vi "Calculate differential torque disproportion.vi"(8 "Error In":errorcluster, 10 "Steering (-123,123)":dbl[unit] format="%#_13g") -> (0 "Error Out":errorcluster, 1 "Right wheel diff scaller":dbl, 2 "Left wheel diff scaller":dbl)   [LabVIEW 2016]
panel:
  out "Right wheel R":dbl[unit]
  out "Left wheel R":dbl[unit]
  out "R xaxis":dbl[unit]
  out "Steer Angle":dbl[unit]
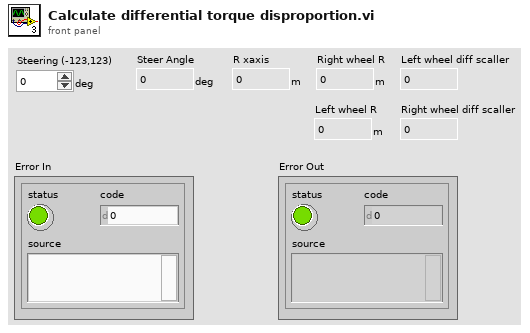
[diagram p1: front panel]
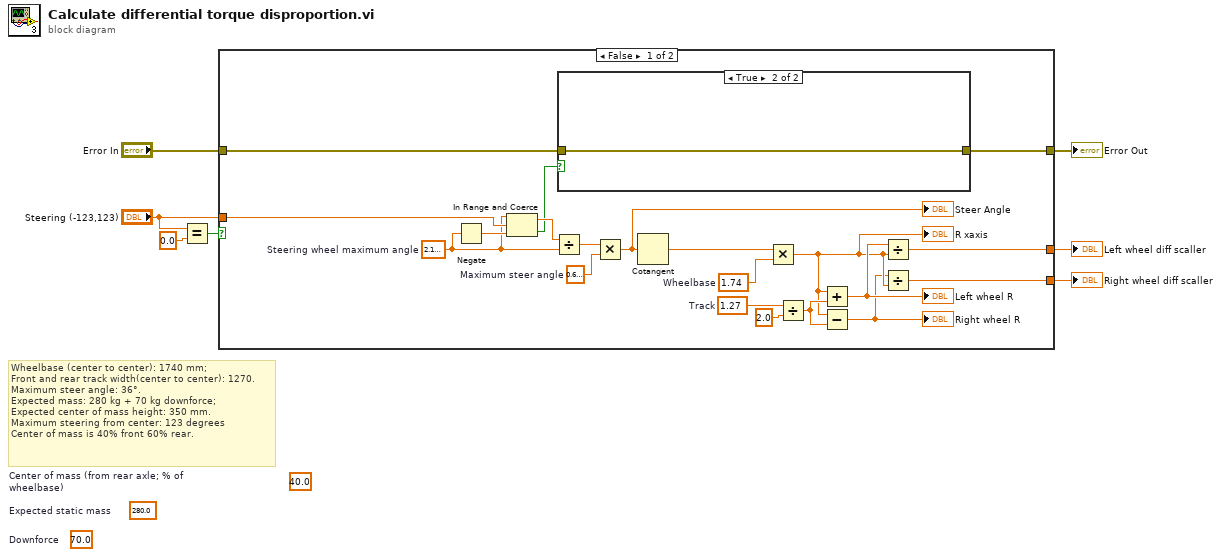
[diagram p0: block diagram]
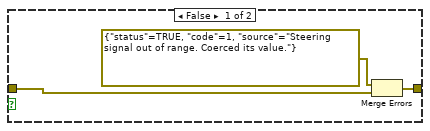
[diagram p2: hidden frame]
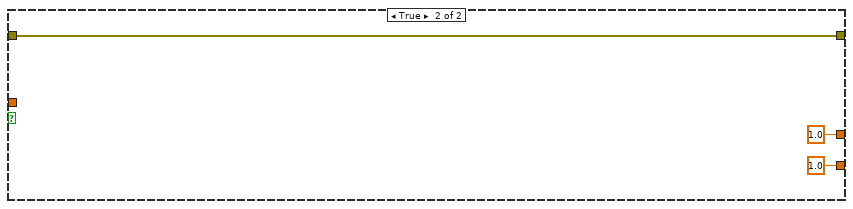
[diagram p3: hidden frame]
diagram:
  (unwired) dbl[unit] 40.0  # Center of mass (from rear axle; % of wheelbase)
  (unwired) dbl[unit] 70.0  # Downforce
  (unwired) dbl[unit] 280.0  # Expected static mass
  # "Wheelbase (center to center): 1740 mm; \nFront and rear track width(center to center): 1270. \nMaximum steer angle: 36°. \nExpected mass: 280 kg + 70 kg downforce; \nExpected center of mass height: 350 mm.\nMaximum steering from center: 123 degrees\nCenter of mass is 40% front 60% rear."
  n1 = Equal?(x="Steering (-123,123)", y=dbl[unit] 0.0) -> (x = y?=w7:bool)
  n2 = case shown="False" w7 {
    tunnel: "Steering (-123,123)" -> [w22 _]
    tunnel: [w24 1.0] -> w4
    tunnel: [w23 1.0] -> w3
    tunnel: "Error In" -> [w9 w32]
    tunnel: [w8 w32] -> w1
    frame False {
      w25 = dbl[unit] 1.27  # Track
      w26 = dbl[unit] 1.74  # Wheelbase
      w27 = dbl[unit] 0.6283185307179586  # Maximum steer angle
      w20 = dbl[unit] 2.1642082724729685  # Steering wheel maximum angle
      n3 = Negate(x=w20) -> (-x=w21:dbl[unit])
      n4 = In Range and Coerce(upper limit=w20, x=w22, lower limit=w21) -> (coerced(x)=w19:dbl[unit], In Range?=w10:bool)
      n5 = Divide(x=w19, y=w20) -> (x/y=w18:dbl)
      n6 = case shown="True" w10 {
        tunnel: w9 -> [w30 w31]
        tunnel: [w29 w31] -> w8
        frame False {
          n7 = Merge Errors(errorcluster {"status"=TRUE, "code"=1, "source"="Steering signal out of range. Coerced its value."} ("error constant"), w30) -> (w29:errorcluster)
        }
        frame True {
        }
      }
      n8 = Multiply(x=w18, y=w27) -> (x*y=w17:dbl[unit])
      "Steer Angle" <- w17
      n9 = Cotangent(1:w17) -> (0:w16:dbl)
      n10 = Multiply(x=w16, y=w26) -> (x*y=w12:dbl[unit])
      "R xaxis" <- w12
      n11 = Divide(x=w25, y=2.0) -> (x/y=w14:dbl[unit])
      n12 = Add(x=w12, y=w14) -> (x+y=w13:dbl[unit])
      "Left wheel R" <- w13
      n13 = Subtract(x=w12, y=w14) -> (x-y=w11:dbl[unit])
      "Right wheel R" <- w11
      n14 = Divide(x=w13, y=w12) -> (x/y=w24:dbl)
      n15 = Divide(x=w11, y=w12) -> (x/y=w23:dbl)
    }
    frame True {
    }
  }
  "Left wheel diff scaller" <- w4
  "Right wheel diff scaller" <- w3
  "Error Out" <- w1
